vi "DesignHighpassFilter.vi"(6 "highpass filter order":i32, 8 "error in (no error)":errorcluster, 9 "highpass cutoff frequency":dbl format="%.2f", 11 "input signal":waveform(sgl)) -> (0 "error out":errorcluster, 2 "IIR Filter Cluster":T1 {"Forward Coefficients" format="%.2f"; "Reverse Coefficients" format="%.2f"}, 3 "dup signal":waveform(sgl))   [LabVIEW 2017, in "CmsVirtualChannel.lvlib"]
uses:
  <vilib>/addons/InsightCM/Devices/Shared/Cms/CmsVirtualChannel/CmsVirtualChannel.lvlib
  <vilib>/Analysis/NI_AALBase.lvlib
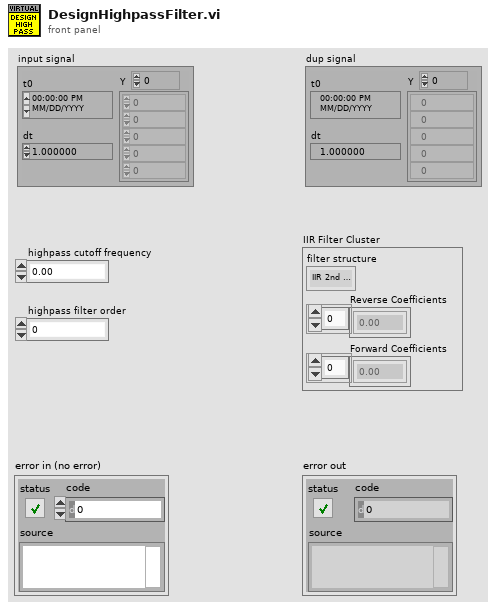
[diagram p1: front panel]
types:
  T1 = cluster{"filter structure":enum32{"IIR 2nd Order", "IIR 4th Order"}, "Reverse Coefficients":dbl[], "Forward Coefficients":dbl[]}
  T2 = enum32{"Lowpass", "Highpass", "Bandpass", "Bandstop"}
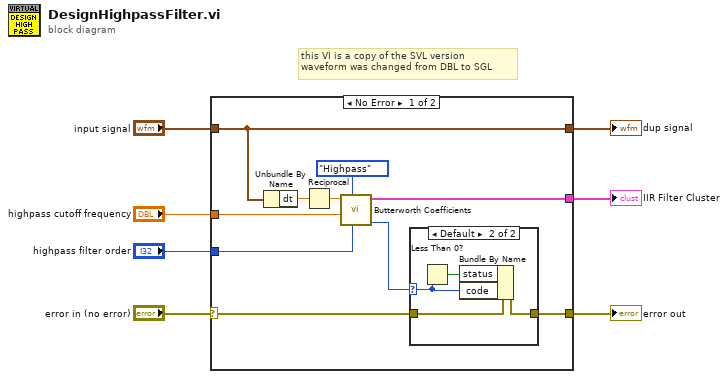
[diagram p0: block diagram]
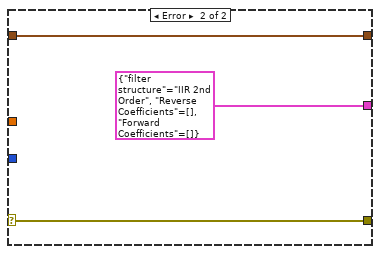
[diagram p3: hidden frame]
diagram:
  # "this VI is a copy of the SVL version\nwaveform was changed from DBL to SGL"
  n1 = case shown="No Error" "error in (no error)" {
    selector: "error in (no error)" -> [w13 w25]
    tunnel: "highpass cutoff frequency" -> [w16 _]
    tunnel: "highpass filter order" -> [w15 _]
    tunnel: [w14 w24] -> w5
    tunnel: "input signal" -> [w14 w24]
    tunnel: [w12 w25] -> w1
    tunnel: [w8 T1 {"filter structure"=enum."IIR 2nd Order", "Reverse Coefficients"=[], "Forward Coefficients"=[]} ("IIR Filter Cluster")] -> w7
    frame No Error {
      n2 = Unbundle By Name(w14) -> ("dt"=w17:dbl)
      n3 = Reciprocal(x=w17) -> (1/x=w9:dbl)
      n4 = call <vilib>:"Butterworth Coefficients.vi"("order"=w15, "filter type"=T2."Highpass", "low cutoff freq: fl"=w16, "sampling freq: fs"=w9) -> ("error"=w11:i32, "IIR Filter Cluster"=w8:T1)  [unwired: 6 in]
      n5 = case shown="Default" w11 {
        selector: w11 -> [_ w20]
        tunnel: w13 -> [w18 w22]
        tunnel: [w18 w21] -> w12
        frame 0 {
        }
        frame Default {
          n6 = Less Than 0?(x=w20) -> (x < 0?=w19:bool)
          n7 = Bundle By Name(cluster=w22, "status"=w19, "code"=w20) -> (w21:errorcluster)
        }
      }
    }
    frame Error {
    }
  }
  "IIR Filter Cluster" <- w7
  "dup signal" <- w5
  "error out" <- w1
